vi "Configure Modules from Hardware.vi"() -> ()   [LabVIEW 2017]
uses:
  NationalInstruments.VeriStand.SystemDefinitionAPI
  <vilib>/addons/VeriStand Custom Device Scripting APIs/SLSC Switch/Scripting/VeriStand SLSC Scripting/VeriStand SLSC Scripting.lvlib
  <vilib>/addons/VeriStand Custom Device Scripting APIs/SLSC Switch/Scripting/SLSC Switch Scripting.lvlib
  SLSC Switch Examples.lvlib
panel:
  in  "SLSC Chassis Name or IP":string
  in  "Controller Name":string
  in  "SLSC Modules":refnum<k21>[](array[refnum])
  in  "Output System Definition file":path
  in  "Input System Definition File":path
  # "Overview: Demonstrates using the SLSC Switch custom device scripting API to configure instances of the custom device to reflect real hardware.\nInstructions:\n1. Browse to the system definition file to be used as input.\n2. Browse to a path to save the system definition file as output.\n3. Set the name of the controller in the system definition file that contains the SLSC Chassis\nand the SLSC Chassis identifier used in the system definition file. \n4. Select the SLSC modules to script into the system definition file.\n5. Run the VI and verify its results."
  # "System Definition Files"
  # "SLSC Chassis"
  # "SLSC Modules"
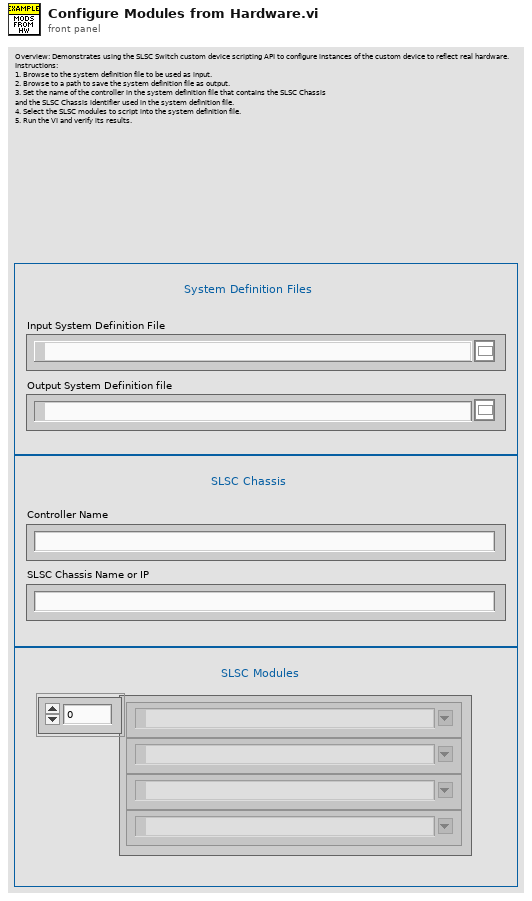
[diagram p1: front panel]
types:
  T1 = typedef "Custom Device API.lvlib/Custom Device Item Ref.ctl" = u64
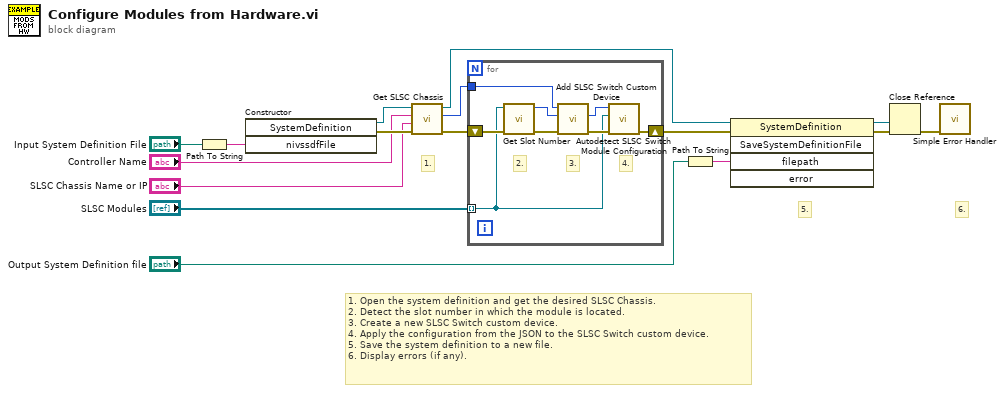
[diagram p0: block diagram]
diagram:
  # "6."
  # "5."
  # "1."
  # "1. Open the system definition and get the desired SLSC Chassis.\n2. Detect the slot number in which the module is located.\n3. Create a new SLSC Switch custom device.\n4. Apply the configuration from the JSON to the SLSC Switch custom device.\n5. Save the system definition to a new file.\n6. Display errors (if any)."
  n1 = Path To String(path="Input System Definition File") -> (string=w9:string)
  n2 = constructor class="SystemDefinition"("nivssdfFile"=w9) -> (reference out=w6:refnum<k24>, error out=w7:errorcluster)  [unwired: 3 in, 2 out]
  n3 = call <vilib>:"Get SLSC Chassis.vi"("error in (no error)"=w7, "SLSC Chassis Name or IP"="SLSC Chassis Name or IP", "Target Name"="Controller Name", "SysDef in"=w6) -> ("error out"=w5:errorcluster, "SLSC Chassis"=w4:u64, "SysDef out"=w3:refnum<k24>)  [unwired: 4 in, 1 out]
  n4 = for {
    tunnel: "SLSC Modules" -> [w17] mode=indexing
    shift-right: [w22] -> w12
    shift-left: w5 -> [w20]
    tunnel: w4 -> [w24]
    # "4."
    # "3."
    # "2."
    n5 = call "Get Slot Number.vi"("error in (no error)"=w20, "SLSC Device"=w17) -> ("error out"=w19:errorcluster, "slot number"=w18:u32)  [unwired: 7 in]
    n6 = call <vilib>:"Add SLSC Switch Custom Device.vi"("error in (no error)"=w19, "Slot Number"=w18, "SLSC Chassis Ref"=w24) -> ("error out"=w23:errorcluster, "SLSC Switch Custom Device Ref"=w21:T1)  [unwired: 6 in, 1 out]
    n7 = call <vilib>:"Autodetect SLSC Switch Module Configuration.vi"("error in"=w23, "SLSC Module"=w17, "SLSC Switch Custom Device Ref in"=w21) -> ("error out"=w22:errorcluster)  [unwired: 7 in, 1 out]
  }
  n8 = Path To String(path="Output System Definition file") -> (string=w16:string)
  n9 = invoke class="SystemDefinition" method="SaveSystemDefinitionFile"(reference=w3, error in=w12, "filepath"=w16) -> (reference out=w14:refnum<k24>, error out=w15:errorcluster)  [unwired: 2 in, 3 out]
  n10 = Close Reference(reference=w14, error in (no error)=w15) -> (error out=w10:errorcluster)
  n11 = call <vilib>:"Simple Error Handler.vi"("error in (no error)"=w10) -> ()  [unwired: 1 in, 8 out]
